vi "Equation of Motion.vi"(0 "effort":dbl[](array[numeric])=[0.0, 0.0, 0.0], 1 "v10":dbl[](array[numeric])=[-1.0, 0.0, 0.0], 2 "v20":dbl[](array[numeric])=[-1.0, 0.0, 0.0], 3 "v30":dbl[](array[numeric])=[-1.0, 0.0, 0.0], 5 "dissipation":dbl[](array[numeric])=[0.0, 0.0, 0.0], 7 "radius":dbl=10.0, 9 "dt":dbl=0.001, 11 "R":T1, 12 "inertia":dbl[](array[numeric])=[0.0, 0.0, 0.0], 14 "flow":dbl[](array[numeric])) -> (4 "v1d":dbl[](array[numeric]) format="%.2f", 6 "v2d":dbl[](array[numeric]) format="%.2f", 8 "v3d":dbl[](array[numeric]) format="%.2f", 10 "R'":T1, 15 "flow'":dbl[](array[numeric]))   [LabVIEW 2017]
uses:
  <vilib>/Analysis/Matrix/Datatypes/RealMatrix.ctl
  <vilib>/Analysis/baseanly.llb/Real A x B.vi
  <vilib>/Analysis/baseanly.llb/A x Vector.vi
  <vilib>/Analysis/_algsub.llb/Vector Norm.vi
  <vilib>/Analysis/_algsub.llb/Real Vector Norm.vi
  <vilib>/Analysis/baseanly.llb/Outer Product.vi
  <vilib>/Analysis/baseanly.llb/Real Outer Product.vi
  <vilib>/robotics/Kinematics/Create Lie Group Matrix.vi
  <vilib>/Analysis/7linalg.llb/Create Special Matrix.vi
  <vilib>/Analysis/7linalg.llb/Create Special Real Matrix.vi
  <vilib>/Analysis/Matrix/Numeric/Multiply/Multiply.vi
  <vilib>/Analysis/Matrix/Numeric/Multiply/Multiply - RM,R.vi
  <vilib>/Analysis/Matrix/Numeric/Multiply/Multiply - R,RM.vi
  <vilib>/Analysis/Matrix/Numeric/Add/Add.vi
  <vilib>/Analysis/Matrix/Numeric/Add/Add - RM,RM.vi
  <vilib>/robotics/Kinematics/NI_Kinematics.lvlib
  <vilib>/Analysis/NI_AALBase.lvlib
  <vilib>/Analysis/Matrix/NI_Matrix.lvlib
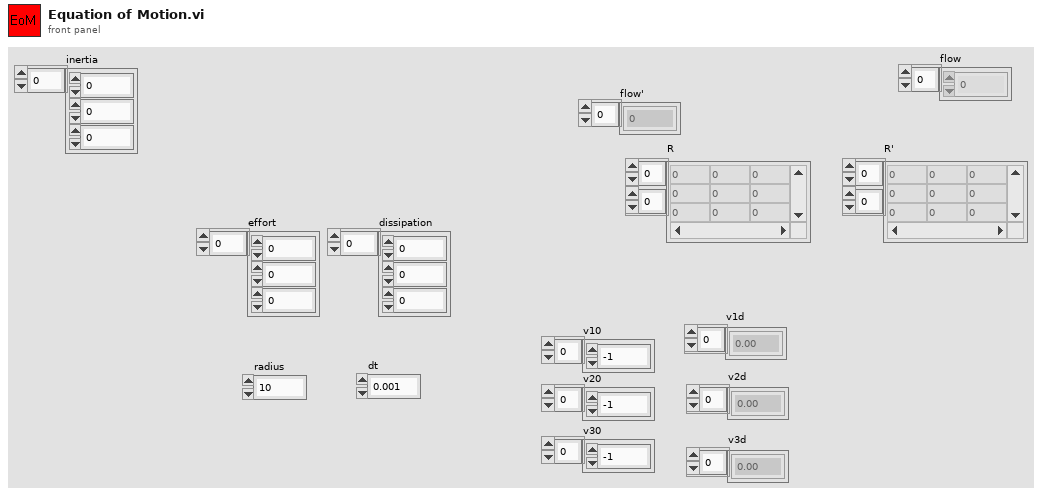
[diagram p1: front panel]
types:
  T1 = typedef "NI_Matrix.lvlib/RealMatrix.ctl" = dbl[][]
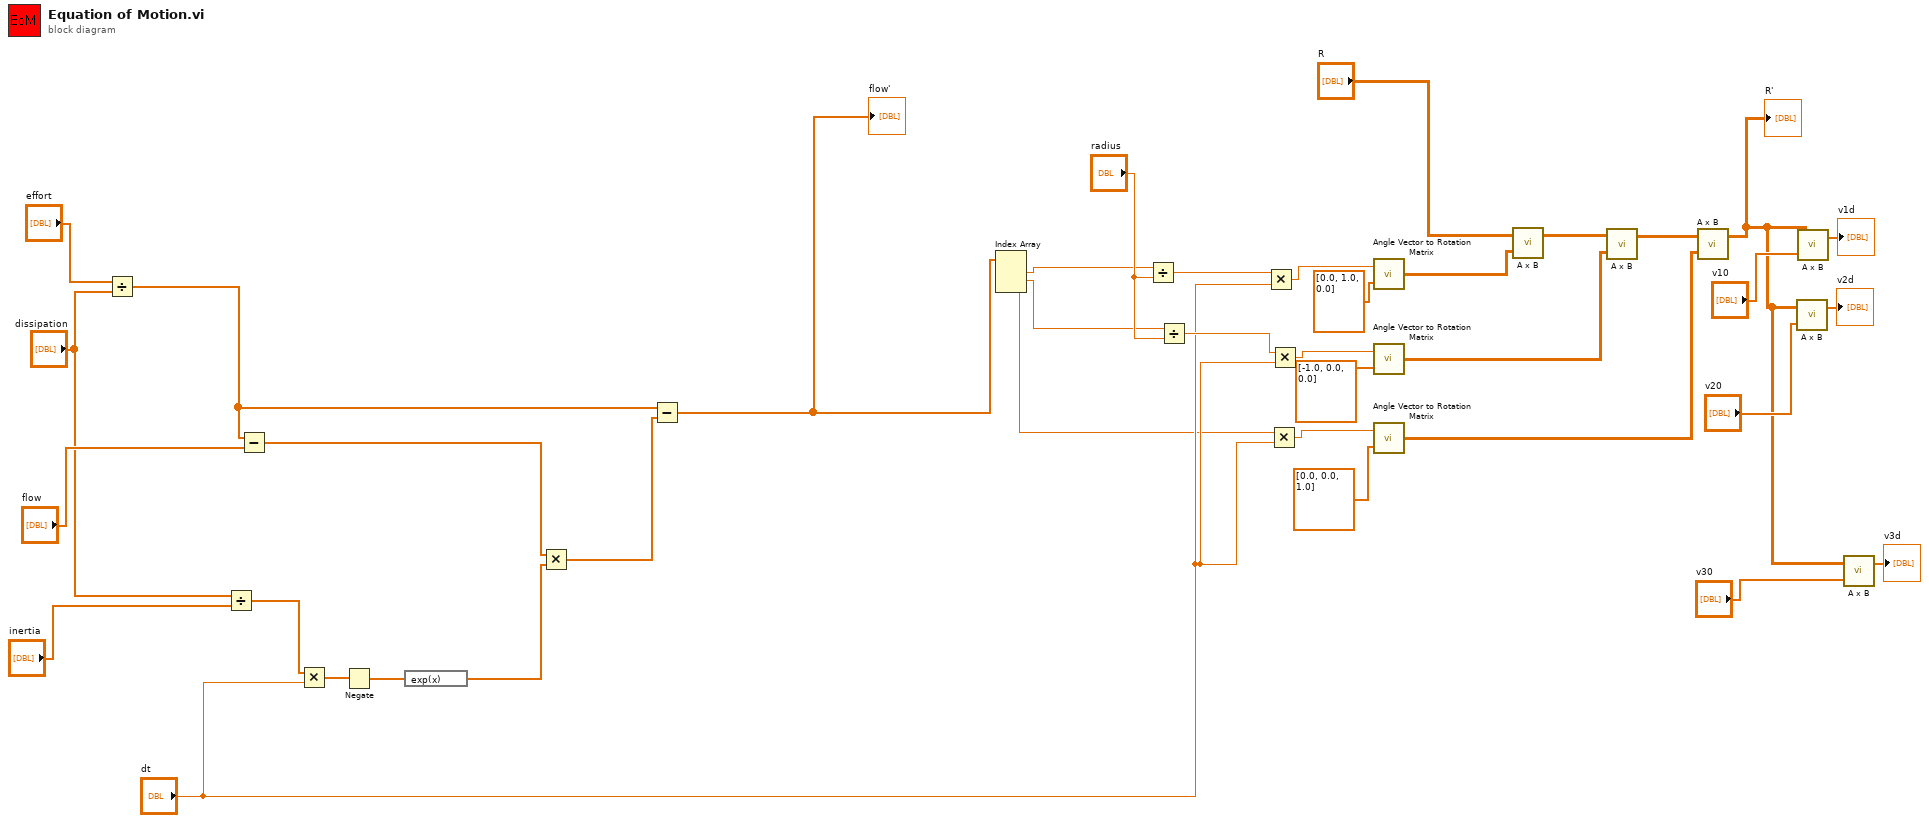
[diagram p0: block diagram]
diagram:
  n1 = Divide(x="effort", y="dissipation") -> (x/y=w6:dbl[])
  n2 = Divide(x="dissipation", y="inertia") -> (x/y=w12:dbl[])
  n3 = Subtract(x=w6, y="flow") -> (x-y=w8:dbl[])
  n4 = Multiply(x=w12, y="dt") -> (x*y=w10:dbl[])
  n5 = Negate(x=w10) -> (-x=w9:dbl[])
  n6 = expression code="exp(x)"(w9) -> (w7:dbl[])
  n7 = Multiply(x=w8, y=w7) -> (x*y=w5:dbl[])
  n8 = Subtract(x=w6, y=w5) -> (x-y=w4:dbl[])
  "flow'" <- w4
  n9 = Index Array(array=w4) -> (element #1=w3:dbl, element #2=w2:dbl, element #3=w1:dbl)  [unwired: 3 in]
  n10 = Divide(x=w3, y="radius") -> (x/y=w36:dbl)
  n11 = Divide(x=w2, y="radius") -> (x/y=w35:dbl)
  n12 = Multiply(x=w36, y="dt") -> (x*y=w34:dbl)
  n13 = Multiply(x=w1, y="dt") -> (x*y=w32:dbl)
  n14 = Multiply(x=w35, y="dt") -> (x*y=w33:dbl)
  n15 = call <vilib>:"Angle Vector to Rotation Matrix.vi"("vector"=dbl[] [0.0, 1.0, 0.0], "angle"=w34) -> ("rotation matrix"=w27:T1)
  n16 = call <vilib>:"Angle Vector to Rotation Matrix.vi"("vector"=dbl[] [-1.0, 0.0, 0.0], "angle"=w33) -> ("rotation matrix"=w25:T1)
  n17 = call <vilib>:"Angle Vector to Rotation Matrix.vi"("vector"=dbl[] [0.0, 0.0, 1.0], "angle"=w32) -> ("rotation matrix"=w23:T1)
  n18 = call-poly <vilib>:"A x B.vi"("B"=w27, "A"="R") -> ("A x B"=w26:T1)  [unwired: 1 out]
  n19 = call-poly <vilib>:"A x B.vi"("B"=w25, "A"=w26) -> ("A x B"=w24:T1)  [unwired: 1 out]
  n20 = call-poly <vilib>:"A x B.vi"("B"=w23, "A"=w24) -> ("A x B"=w20:T1)  [unwired: 1 out]
  "R'" <- w20
  n21 = call-poly <vilib>:"A x B.vi"("Vector"="v20", "A"=w20) -> ("A x Vector"=→"v2d":dbl[])  [unwired: 1 out]
  n22 = call-poly <vilib>:"A x B.vi"("Vector"="v10", "A"=w20) -> ("A x Vector"=→"v1d":dbl[])  [unwired: 1 out]
  n23 = call-poly <vilib>:"A x B.vi"("Vector"="v30", "A"=w20) -> ("A x Vector"=→"v3d":dbl[])  [unwired: 1 out]
